vi "force_clamp_v3.vi"(2 "reinitialize? (F) 2":bool, 4 "handle in":i32, 6 "Pos 0":dbl, 7 "Desired Force (pN)":dbl, 8 "error in (no error)":errorcluster, 9 "QPD":dbl, 10 "Apply Force":bool, 11 "Nanostage":dbl) -> (0 "error out":errorcluster, 3 "QPD delta":dbl)   [LabVIEW 2019]
uses:
  <vilib>/addons/control/pid/pid.llb/PID (DBL).vi
  <vilib>/addons/control/pid/NI_PID_pid.lvlib
  Program Files/Mad City Labs/NanoDrive/Labview Examples/Madlib.dll
panel:
  in  "dt (s)":dbl=-1.0 format="%.3f"
  out "Setpoint":dbl
  in  "output range":cluster{"output high":dbl, "output low":dbl}={"output high"=0.1, "output low"=-0.1} {"output low" format="%.2f"; "output high" format="%.2f"}
  out "PID output":dbl format="%.2f"
  in  "PID gains":T1={"proportional gain (Kc)"=0.5, "integral time (Ti, min)"=0.0, "derivative time (Td, min)"=0.0} {"derivative time (Td, min)" min=-1e-18 max=1000000000000000.0 step=1e-05 format="%.3f"; "integral time (Ti, min)" min=-1e-18 step=1e-05 format="%.6f"; "proportional gain (Kc)" min=-1e-18 step=1e-05 format="%.5f"}
  # "PID for holding a tethered DNA molecule ata constant force, determined by the BT value of the QPD.\nThe code is mainly inspired by the PID example VI shipped with LabVIEW. See it for further details."
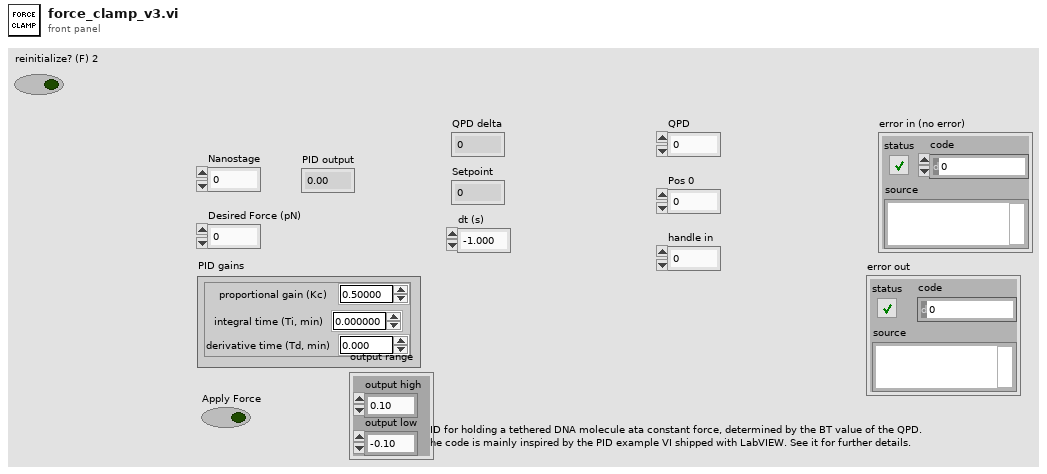
[diagram p1: front panel]
types:
  T1 = cluster{"proportional gain (Kc)":dbl, "integral time (Ti, min)":dbl, "derivative time (Td, min)":dbl}
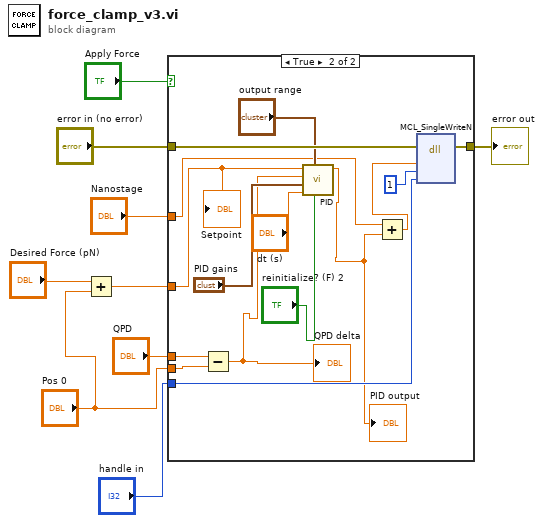
[diagram p0: block diagram]
diagram:
  n1 = Add(x="Desired Force (pN)", y="Pos 0") -> (x+y=w1:dbl)
  n2 = case shown="True" "Apply Force" {
    tunnel: "QPD" -> [_ w25]
    tunnel: "Pos 0" -> [_ w22]
    tunnel: w1 -> [_ w21]
    tunnel: "Nanostage" -> [_ w15]
    tunnel: "handle in" -> [_ w20]
    tunnel: "error in (no error)" -> [w10 w19]
    tunnel: [w10 w18] -> w4
    frame False {
    }
    frame True {
      n3 = Subtract(x=w25, y=w22) -> (x-y=w14:dbl)
      "QPD delta" <- w14
      n4 = call-poly <vilib>:"PID.vi"("reinitialize? (F)"="reinitialize? (F) 2", "output range"="output range", "dt (s)"="dt (s)", "PID gains"="PID gains", "process variable"=w14, "setpoint"=w21) -> ("output"=w12:dbl)  [unwired: 4 in, 1 out]
      "PID output" <- w12
      n5 = Add(x=w15, y=w12) -> (x+y=w16:dbl)
      n6 = dll-call lib="C:/Program Files/Mad City Labs/NanoDrive/Labview Examples/MADLib.dll" fn="MCL_SingleWriteN"(error in=w19, "position"=w16, "axis"=u32 1, "handle"=w20) -> (error out=w18:errorcluster)  [unwired: 6 in, 1 out]
      "Setpoint" <- w21
    }
  }
  "error out" <- w4
